vi "DatabaseTest.vi"(3 "error in (no error)":errorcluster, 5 "联机模式":enum16{"单机", "追溯"}(ring)) -> (0 "error out":errorcluster, 2 "数据库连接成功":bool)   [LabVIEW 2020]
uses:
  <vilib>/Utility/error.llb/DialogType.ctl
  <vilib>/addons/database/Connection.llb/DB Tools Open Connec (String).vi
  <vilib>/addons/database/NI_Database_API.lvlib
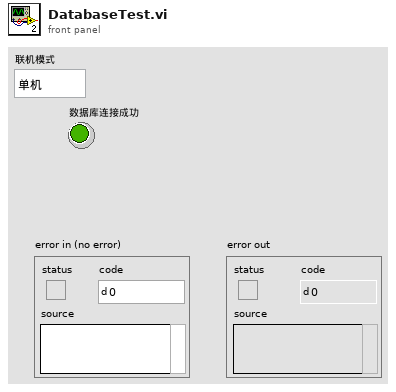
[diagram p1: front panel]
types:
  T1 = typedef "DialogType.ctl" = u16
  T2 = typedef "NI_Database_API.lvlib/Conn ObjectReference.ctl" = refnum<k1>
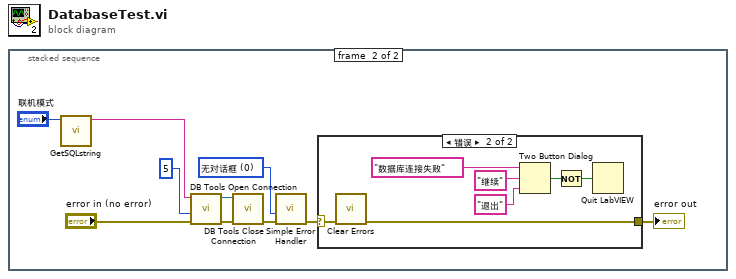
[diagram p0: block diagram]
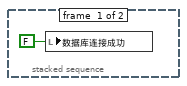
[diagram p2: hidden frame]
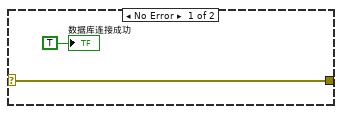
[diagram p3: hidden frame]
diagram:
  n1 = stacked-sequence {
    frame #0 {
      n2 = local write "数据库连接成功"(FALSE ("数据库连接成功")) -> ()
    }
    frame #1 {
      w7 = T1 0 items=["无对话框", "确定信息", "继续或停止信息", "确定信息＋警告", "继续/停止+警告"] ("type of dialog (OK msg:1)")
      n3 = call "GetSQLstring.vi"("联机模式"="联机模式") -> ("连接字符串"=w3:string)  [unwired: 9 in, 1 out]
      n4 = call-poly <vilib>:"DB Tools Open Connection.vi"("error in (no error)"="error in (no error)", "connection timeout (15)"=5, "connection information"=w3) -> ("error out"=w11:errorcluster, "connection reference"=w10:T2)  [unwired: 5 in]
      n5 = call <vilib>:"DB Tools Close Connection.vi"("error in (no error)"=w11, "connection reference"=w10) -> ("error out"=w8:errorcluster)  [unwired: 5 in]
      n6 = call <vilib>:"Simple Error Handler.vi"("type of dialog (OK msg:1)"=w7, "error in (no error)"=w8) -> ("error out"=w5:errorcluster)  [unwired: 3 in, 4 out]
      n7 = case shown="错误" w5 {
        selector: w5 -> [w12 w15]
        tunnel: [w12 w14] -> w4
        frame No Error {
          "数据库连接成功" <- TRUE ("数据库连接成功")
        }
        frame Error {
          n8 = call <vilib>:"Clear Errors.vi"("error in (no error)"=w15) -> ("error out"=w14:errorcluster)  [unwired: 5 in, 1 out]
          n9 = Two Button Dialog(message="数据库连接失败" ("消息"), 1:"退出" ("F按钮名称（“取消”）"), 2:"继续" ("T按钮名称（“确定”）")) -> (T button?=w17:bool)
          n10 = Not(x=w17) -> (.not. x?=w16:bool)
          n11 = Quit LabVIEW(quit? (T)=w16) -> ()
        }
      }
      "error out" <- w4
    }
  }
